vi "Read Text.vi"(6 "timeout ms (5000)":i32=5000, 8 "error in (no error)":errorcluster, 9 "RawSocket Handler in":refnum<class "RawSocket Handler.lvclass">) -> (1 "String":string, 2 "error out":errorcluster, 3 "RawSocket Handler out":refnum<class "RawSocket Handler.lvclass">)   [LabVIEW 2020, in "wamplv.lvlib" / "RawSocket Handler.lvclass"]
uses:
  RawSocket Handler.lvclass
  RawSocket Handler.lvclass/RawSocket Handler.ctl
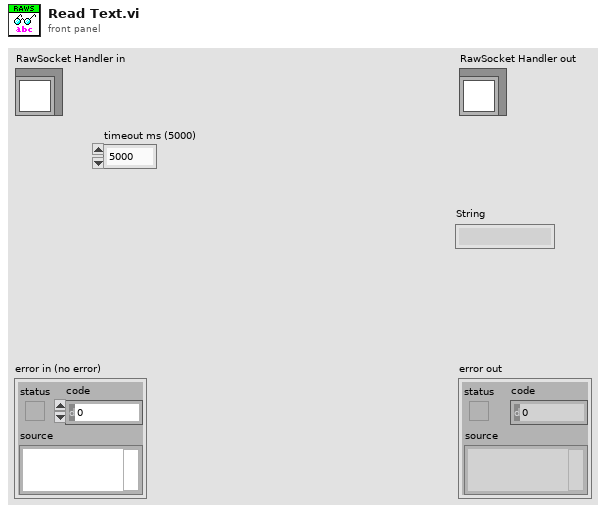
[diagram p1: front panel]
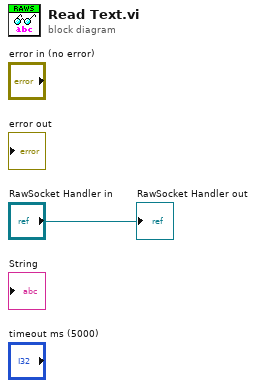
[diagram p0: block diagram]
diagram:
  "RawSocket Handler out" <- "RawSocket Handler in"
